vi "Main.vi"(11 "Module Admin":refnum<class "Delacor_lib_QMH_Module Admin.lvclass">) -> ()   [LabVIEW 2020, in "Motherboard loading.lvlib"]
doc: "This template is based off of the Queued Message Handler design pattern and the Queued Message Handler project template that ships with LabVIEW.\n\nThe main difference is that the queue is private to this module and communication between modules is performed via Broadcast and Request events.\n\nRequest events are wrapped in public API methods and are handled in the Event Handling Loop (EHL) of this VI. Any module can register for Broadcast events sent by this module. The EHL generates messages based on user interface actions.\n\nThe Message Handling Loop (MHL) processes messages generated by the EHL, or by other messages. The messages are string values, so new messages can be added easily to the Message Cases case structure in the MHL. Each message cluster can also provide an optional value for Message Data, which is a variant that can be converted to whatever message-specific data is required.\n_____\nBased on DQMH Project Template 6.1.0.94."
uses:
  Motherboard loading.lvlib
  <vilib>/Delacor/Delacor QMH/Libraries/Module Admin_class/Delacor_lib_QMH_Module Admin.lvclass
  Module Data--cluster.ctl
  <vilib>/Delacor/Delacor QMH/Libraries/Message Queue_class/Delacor_lib_QMH_Message Queue.lvclass/Delacor_lib_QMH_Message Queue.ctl
  Stop Argument--cluster.ctl
  <vilib>/Delacor/Delacor QMH/Libraries/Module Admin_class/Delacor_lib_QMH_Module Admin.lvclass/Delacor_lib_QMH_Module Admin.ctl
  Start acquisition Argument--cluster.ctl
  Start acquisition (Reply Payload)--cluster.ctl
  Stop acquisition Argument--cluster.ctl
  System.Management
  <vilib>/Utility/miscctls.llb/LVPointTypeDef.ctl
  <vilib>/Delacor/Delacor QMH/Libraries/Message Queue_class/Delacor_lib_QMH_Enqueue Message (Single).vi
  <vilib>/Delacor/Delacor QMH/Libraries/Module Admin_class/Delacor_lib_QMH_Get External Launch.vi
  <vilib>/Utility/error.llb/Error Cluster From Error Code.vi
  <vilib>/ErrorRing/Error Ring.xnode
  <vilib>/Delacor/Delacor QMH/Libraries/Message Queue_class/Delacor_lib_QMH_Message Queue.lvclass
panel:
  in  "format":i32(ring) items=["Mof", "CimDtd20", "WmiDtd20"]
  out "error out":errorcluster
  out "Status":string
  in  "Simulate MHL Error":bool
  in  "Simulate EHL Error":bool
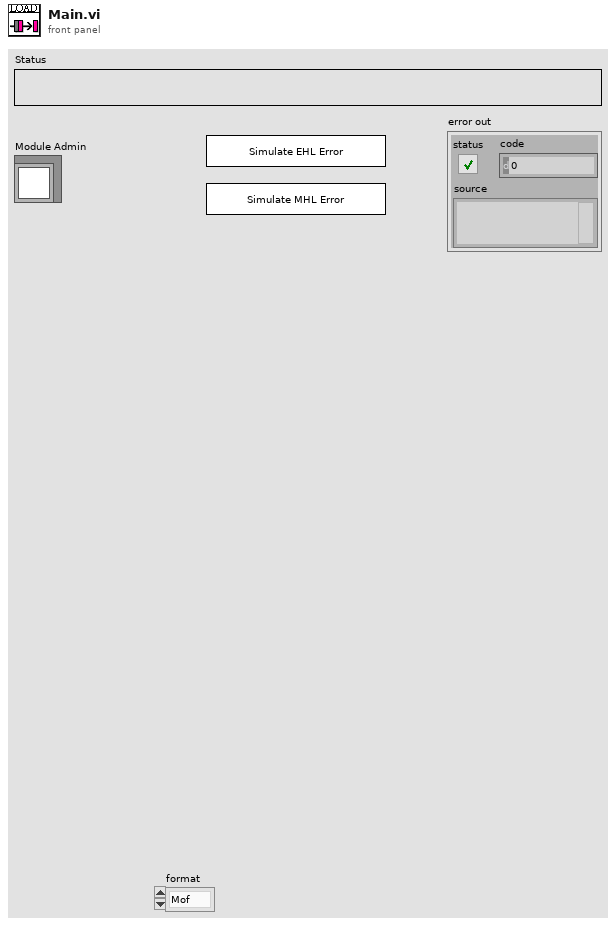
[diagram p1: front panel]
types:
  T1 = typedef "Motherboard loading.lvlib/Request Events--cluster.ctl" = cluster{"Stop Module":refnum<user-event>, "Show Panel":refnum<user-event>, "Hide Panel":refnum<user-event>, "Get Module Execution Status":refnum<user-event>, "Show Diagram":refnum<user-event>, "Start acquisition":refnum<user-event>, "Wake up Load detect HL":refnum<user-event>, "Put Load update HL to sleep":refnum<user-event>, "Stop acquisition":refnum<user-event>}
  T2 = typedef "Motherboard loading.lvlib/Module Data--cluster.ctl" = cluster{"Status":string}
  T3 = enum32{"invalid lock state", "Not Locked", "Locked (No Password)", "Password-protected"}
  T4 = typedef "Motherboard loading.lvlib/Stop Argument--cluster.ctl" = cluster{"Origin":string, "Exit via Stop Module Req?":bool, "Wait for Module to stop?":bool}
  T5 = typedef "Motherboard loading.lvlib/Start acquisition Argument--cluster.ctl" = cluster{"Boolean":bool, "Wait Notifier":refnum<notifier>, "wait for reply":bool, "Detecting speed":dbl}
  T6 = typedef "Motherboard loading.lvlib/Stop acquisition Argument--cluster.ctl" = cluster{"Boolean":bool}
  T7 = typedef "LVPointTypeDef.ctl" = cluster{"Horizontal":i16, "Vertical":i16}
  T8 = enum32{"Invalid", "Standard", "Closed", "Hidden", "Minimized", "Maximized"}
  T9 = typedef "Motherboard loading.lvlib/Start acquisition (Reply Payload)--cluster.ctl" = cluster{"error":errorcluster}
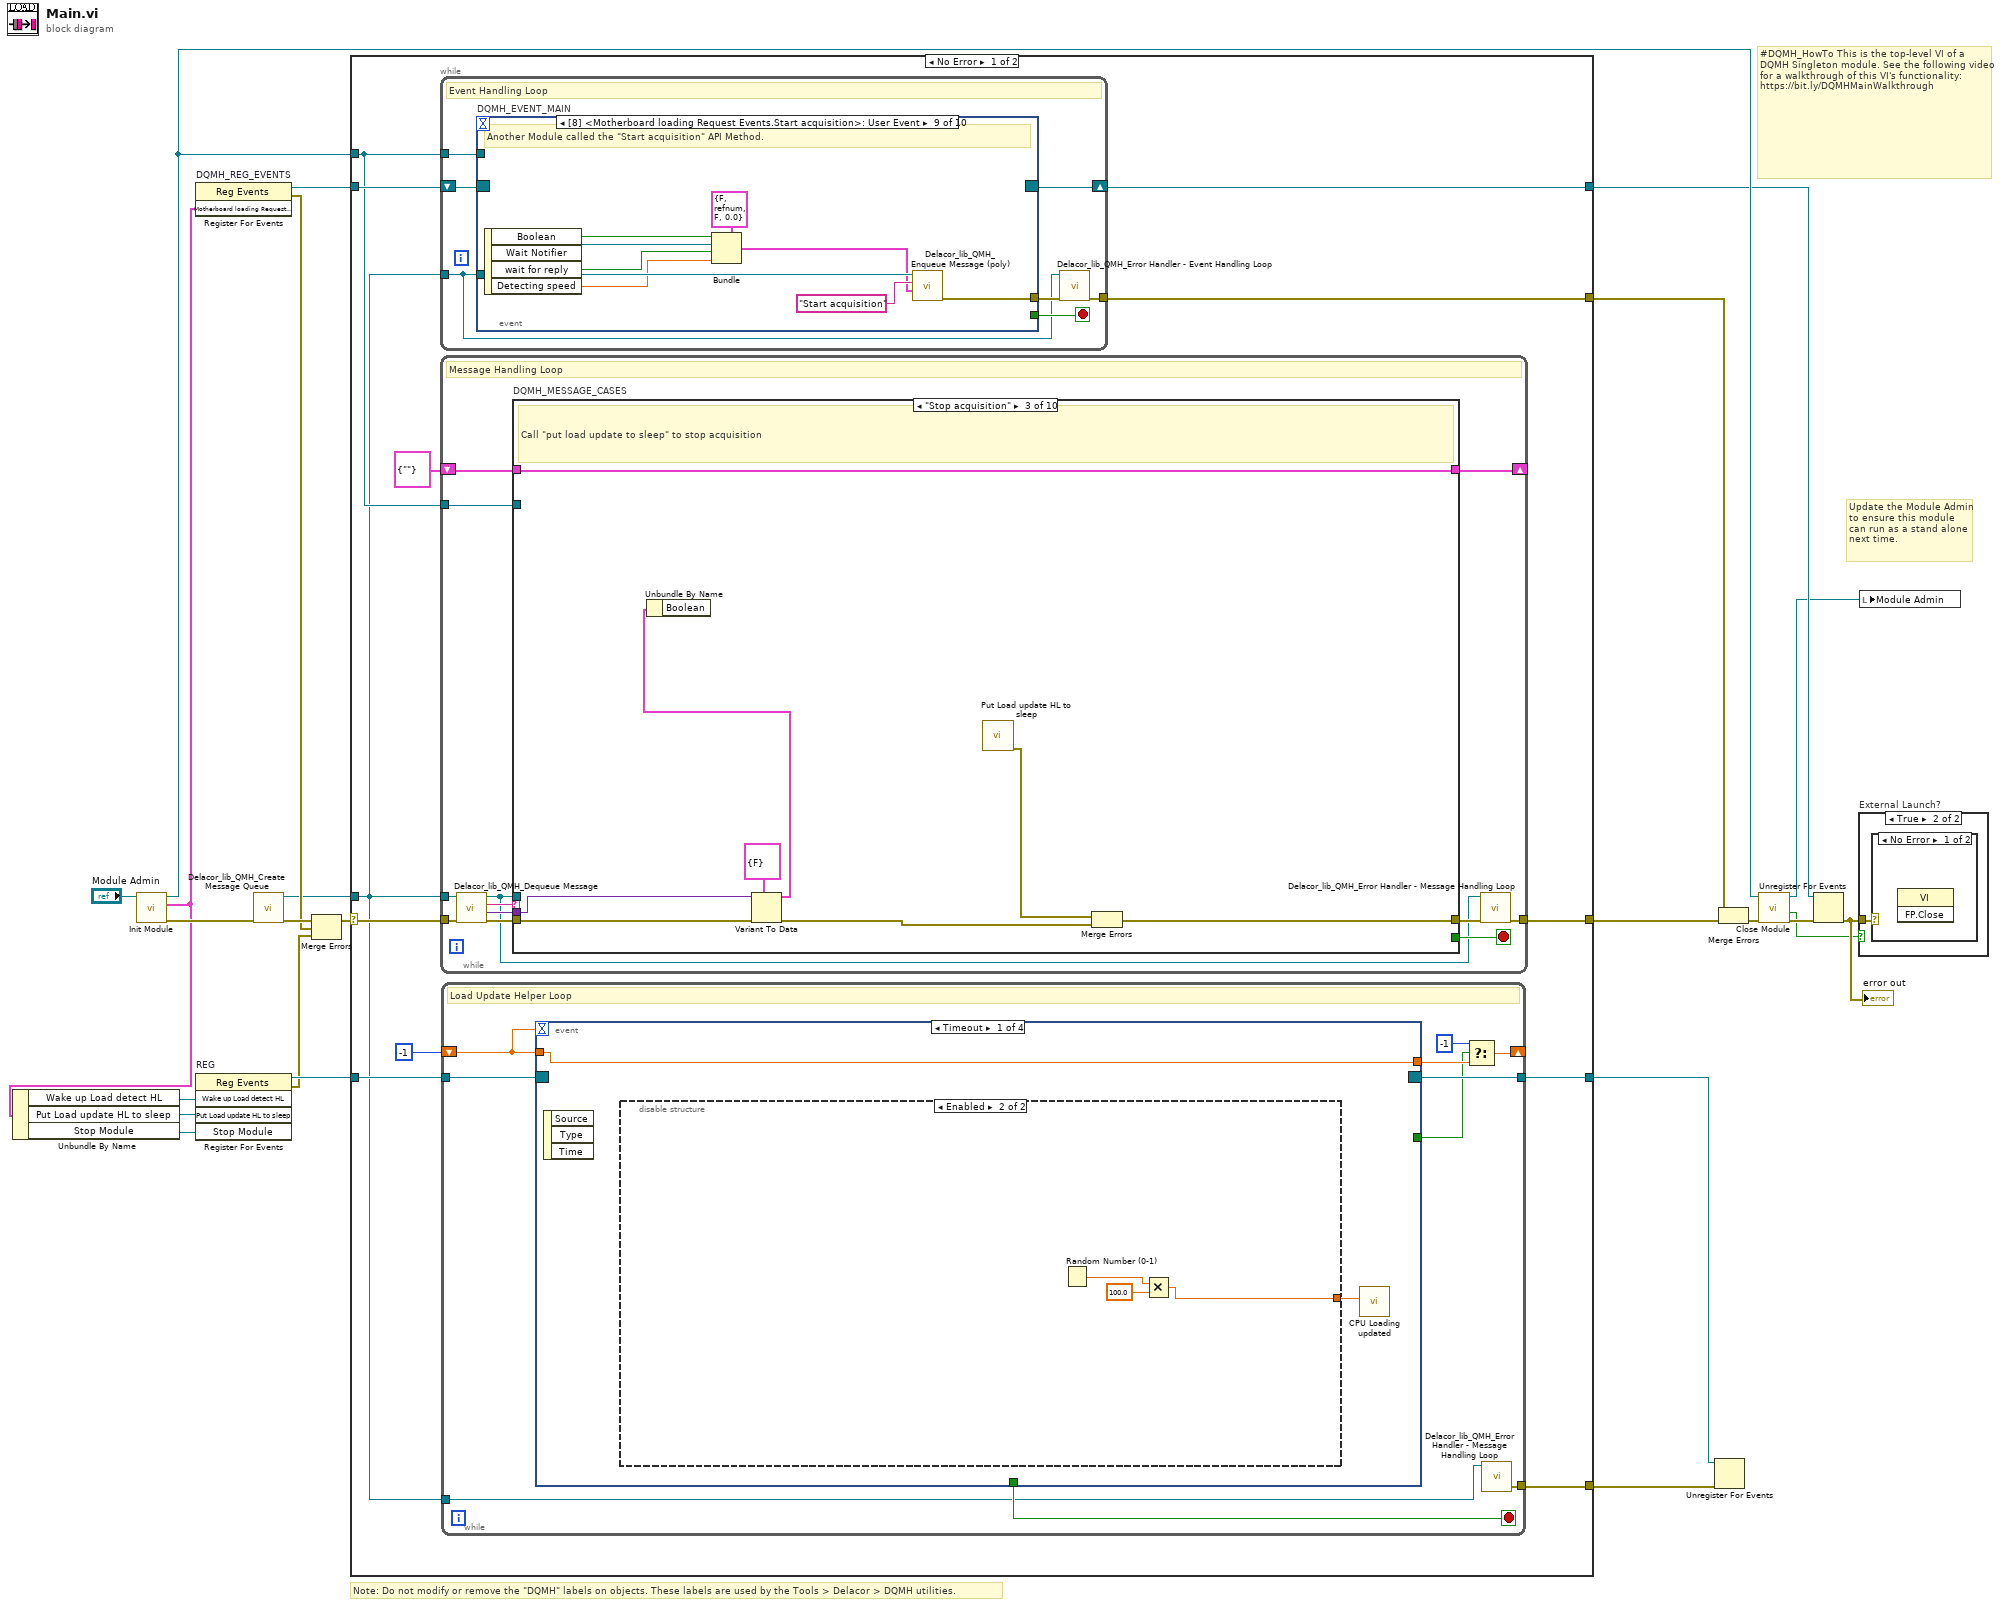
[diagram p0: block diagram]
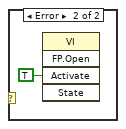
[diagram p3: hidden frame]
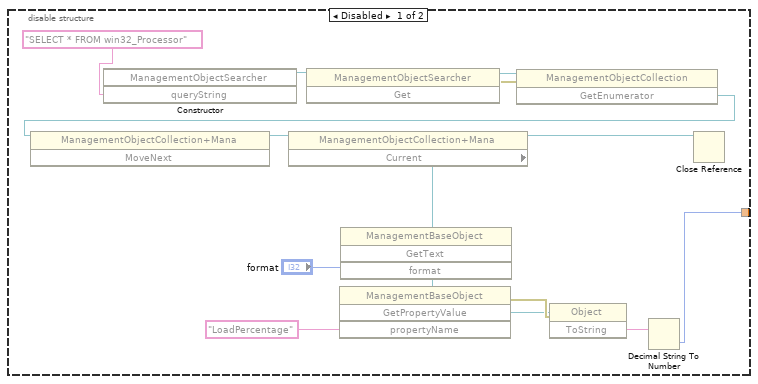
[diagram p4: hidden frame]
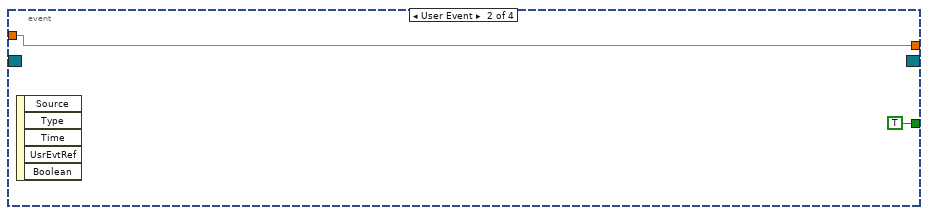
[diagram p5: hidden frame]
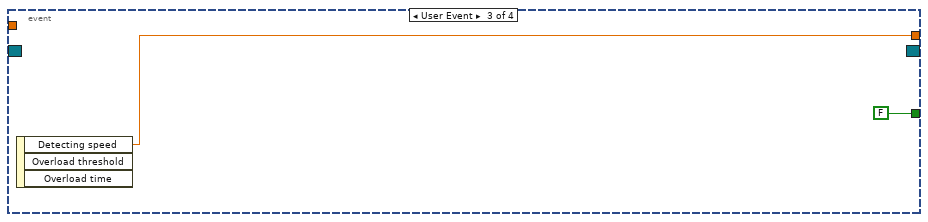
[diagram p6: hidden frame]
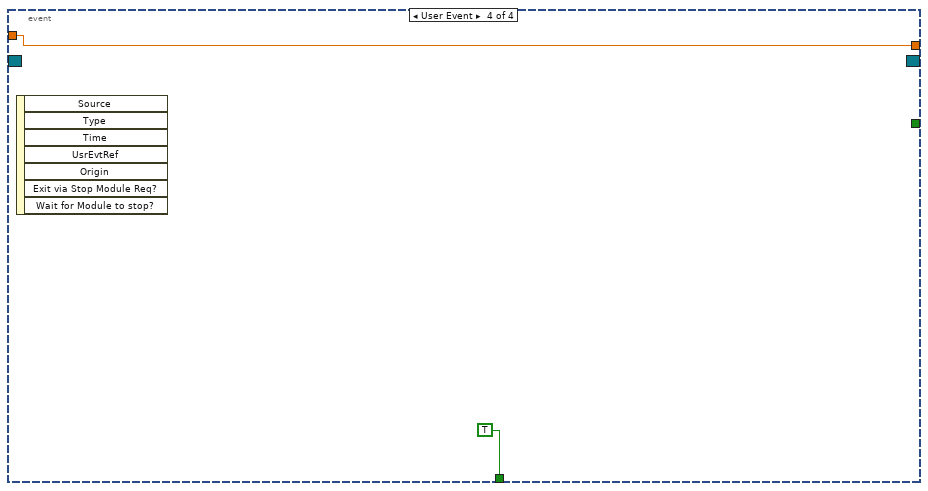
[diagram p7: hidden frame]
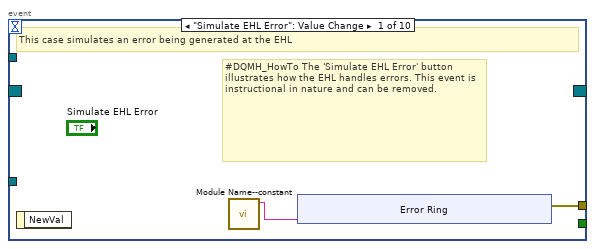
[diagram p8: hidden frame]
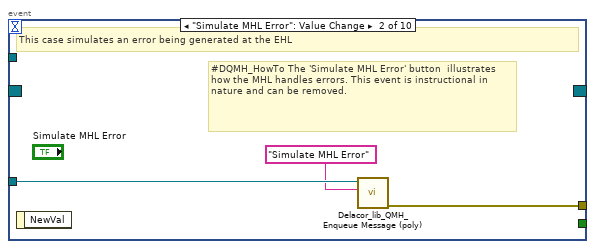
[diagram p9: hidden frame]
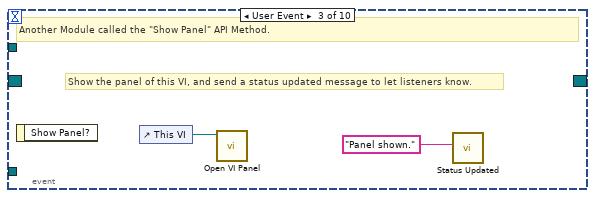
[diagram p10: hidden frame]
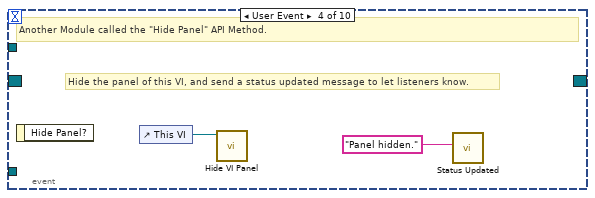
[diagram p11: hidden frame]
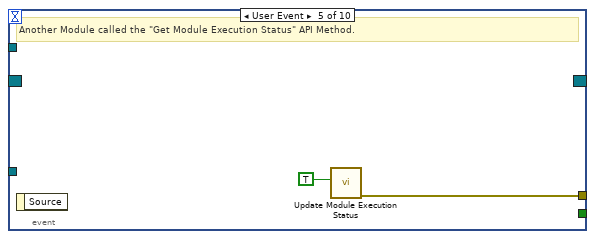
[diagram p12: hidden frame]
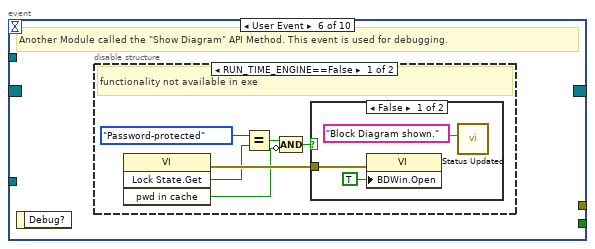
[diagram p13: hidden frame]
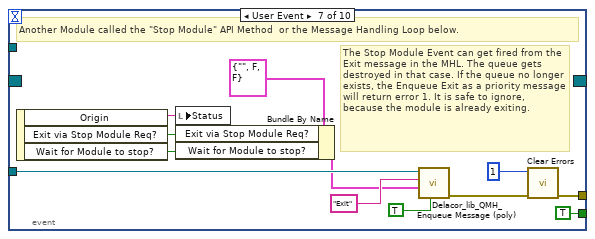
[diagram p16: hidden frame]
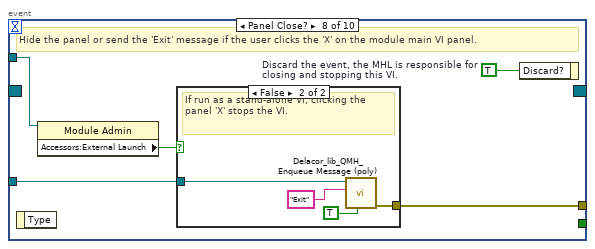
[diagram p17: hidden frame]
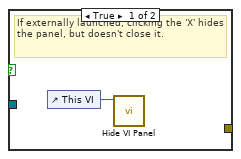
[diagram p18: hidden frame]
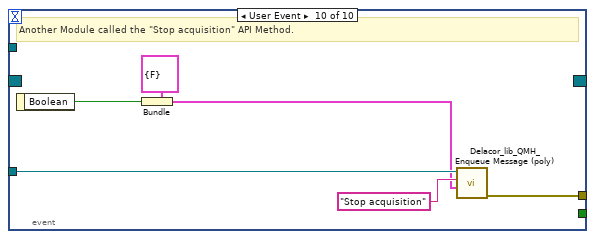
[diagram p19: hidden frame]
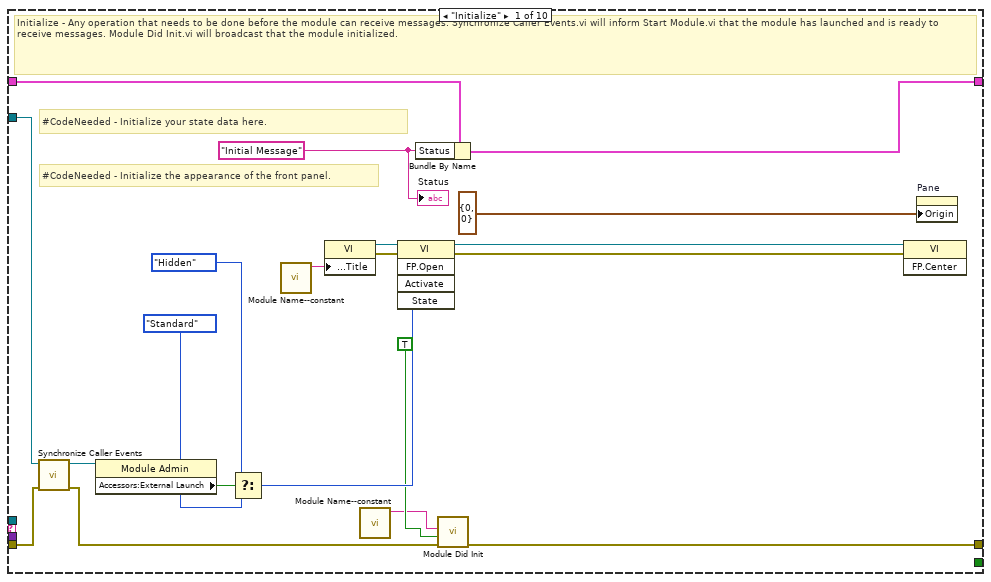
[diagram p20: hidden frame]
diagram:
  # "#DQMH_HowTo This is the top-level VI of a DQMH Singleton module. See the following video for a walkthrough of this VI's functionality: https://bit.ly/DQMHMainWalkthrough"
  # "Note: Do not modify or remove the \"DQMH\" labels on objects. These labels are used by the Tools > Delacor > DQMH utilities."
  # "Update the Module Admin to ensure this module can run as a stand alone next time."
  n1 = call "Init Module.vi"("Singleton Module Admin in"="Module Admin") -> ("error out"=w23:errorcluster, "Motherboard loading Request Events"=w2:T1, "Singleton Module Admin out"=w15:refnum<class "Delacor_lib_QMH_Module Admin.lvclass">)  [unwired: 8 in]
  n2 = Unbundle By Name(w2) -> ("Wake up Load detect HL"=w5:refnum<user-event>, "Put Load update HL to sleep"=w4:refnum<user-event>, "Stop Module"=w3:refnum<user-event>)
  n3 = register-events "DQMH_REG_EVENTS"(w2) -> (reference out=w13:refnum<event-registration>, error out=w16:errorcluster)  [unwired: 2 in]
  n4 = register-events "REG"(w5, w4, w3) -> (reference out=w8:refnum<event-registration>, error out=w1:errorcluster)  [unwired: 2 in]
  n5 = call <vilib>:"Delacor_lib_QMH_Create Message Queue.vi"("error in"=w23) -> ("error out"=w18:errorcluster, "Message Queue"=w12:refnum<class "Delacor_lib_QMH_Message Queue.lvclass">)  [unwired: 9 in]
  n6 = Merge Errors(w18, w16, w1) -> (w17:errorcluster)
  n7 = case shown="No Error" w17 {
    selector: w17 -> [w34 w267]
    tunnel: [w36 w266] -> w24
    tunnel: [w33 w272] -> w14
    tunnel: w13 -> [w31 w272]
    tunnel: w12 -> [w26 w265]
    tunnel: [w35 _] -> w21
    tunnel: w15 -> [w30 w268]
    tunnel: w8 -> [w29 w264]
    tunnel: [w28 _] -> w7
    tunnel: [w27 w264] -> w6
    frame No Error {
      n8 = while {
        tunnel: w26 -> [w72]
        shift-right: [w75] -> w33
        shift-left: w31 -> [w76]
        tunnel: [w77] -> w35
        tunnel: w30 -> [w73]
        stop <- w74 stop-if-true
        # "Event Handling Loop"
        n9 = event "DQMH_EVENT_MAIN" shown="[8] <Motherboard loading Request Events.Start acquisition>: User Event" {
          selector: w76 -> [_ _ _ _ _ _ _ _ _ _]
          dyn-events: [_ _ _ _ _ _ _ _ _ _] -> w75
          timeout: _ -> [_ _ _ _ _ _ _ _ _ _]
          tunnel: [_ _ _ _ _ _ TRUE ("Discard?") _ _ _] -> w74
          tunnel: w72 -> [_ w89 _ _ _ _ w113 w120 w136 w142]
          tunnel: [w80 w90 _ _ w96 _ w116 w122 w132 w137] -> w78
          tunnel: w73 -> [_ _ _ _ _ _ _ w119 _ _]
          event "Simulate EHL Error": Value Change {
            # "#DQMH_HowTo The 'Simulate EHL Error' button  illustrates how the EHL handles errors. This event is instructional in nature and can be removed."
            # "This case simulates an error being generated at the EHL"
            n10 = event-data() -> ()  [unwired: 1 in, 1 out]
            n11 = call "Module Name--constant.vi"() -> ("Module Name"=w79:string)  [unwired: 11 in]
            n12 = xnode "Error Ring"("parameter 0"=w79) -> ("error out"=w80:errorcluster)
          }
          event "Simulate MHL Error": Value Change {
            # "#DQMH_HowTo The 'Simulate MHL Error' button  illustrates how the MHL handles errors. This event is instructional in nature and can be removed."
            # "This case simulates an error being generated at the EHL"
            n13 = event-data() -> ()  [unwired: 1 in, 1 out]
            n14 = call-poly <vilib>:"Delacor_lib_QMH_Enqueue Message (poly).vi"("Message"="Simulate MHL Error", "Message Queue in"=w89) -> ("error out"=w90:errorcluster)  [unwired: 8 in, 1 out]
          }
          event User Event {
            # "Show the panel of this VI, and send a status updated message to let listeners know."
            # "Another Module called the \"Show Panel\" API Method."
            n15 = event-data() -> ()  [unwired: 1 in, 1 out]
            n16 = control-ref of="This VI"() -> (w92:refnum<vi>)
            n17 = call "Open VI Panel.vi"("VI"=w92) -> ()  [unwired: 10 in, 1 out]
            n18 = call "Status Updated.vi"("Status"="Panel shown." ("format string")) -> ()  [unwired: 10 in, 1 out]
          }
          event User Event {
            # "Hide the panel of this VI, and send a status updated message to let listeners know."
            # "Another Module called the \"Hide Panel\" API Method."
            n19 = event-data() -> ()  [unwired: 1 in, 1 out]
            n20 = control-ref of="This VI"() -> (w94:refnum<vi>)
            n21 = call "Hide VI Panel.vi"("VI"=w94) -> ()  [unwired: 10 in, 1 out]
            n22 = call "Status Updated.vi"("Status"="Panel hidden." ("format string")) -> ()  [unwired: 10 in, 1 out]
          }
          event User Event {
            # "Another Module called the \"Get Module Execution Status\" API Method."
            n23 = event-data() -> ()  [unwired: 1 in, 1 out]
            n24 = call "Update Module Execution Status.vi"("Running?"=TRUE) -> ("error out"=w96:errorcluster)  [unwired: 10 in]
          }
          event User Event {
            # "Another Module called the \"Show Diagram\" API Method. This event is used for debugging."
            n25 = event-data() -> ()  [unwired: 1 in, 1 out]
            n26 = disable-structure shown="RUN_TIME_ENGINE==False" {
              frame condition #0 (active) {
                # "functionality not available in exe"
                n27 = invoke class="VI" method="Lock State.Get"() -> (error out=w102:errorcluster, "Get Lock State"=w101:T3, "pwd in cache"=w98:bool)  [unwired: 4 in, 1 out]
                n28 = Equal?(x=T3."Password-protected", y=w101) -> (x = y?=w99:bool)
                n29 = Compound Arithmetic op=AND(w99, invert w98) -> (w97:bool)
                n30 = case shown="False" w97 {
                  tunnel: w102 -> [w105 _]
                  frame False {
                    n31 = property class="VI"(error in=w105, "BDWin.Open"=TRUE ("Block Diagram Window:Open")) -> ()  [unwired: 1 in, 2 out]
                    n32 = call "Status Updated.vi"("Status"="Block Diagram shown." ("format string")) -> ()  [unwired: 10 in, 1 out]
                  }
                  frame True {
                    # "Password-protected VI, and the password is not in the cache. Do not show the diagram."
                  }
                }
              }
              frame condition #1 {
              }
            }
          }
          event User Event {
            # "The Stop Module Event can get fired from the Exit message in the MHL. The queue gets destroyed in that case. If the queue no longer exists, the Enqueue Exit as a priority message will return error 1. It is safe to ignore, because the module is already exiting."
            # "Another Module called the \"Stop Module\" API Method  or the Message Handling Loop below."
            n33 = event-data() -> ("Origin"=w112:string, "Exit via Stop Module Req?"=w108:bool, "Wait for Module to stop?"=w107:bool)  [unwired: 1 in]
            n34 = local write "Status"(w112) -> ()
            n35 = Bundle By Name(cluster=T4 {"Origin"="", "Exit via Stop Module Req?"=FALSE, "Wait for Module to stop?"=FALSE} ("Stop Argument"), "Exit via Stop Module Req?"=w108, "Wait for Module to stop?"=w107) -> (w106:T4)
            n36 = call-poly <vilib>:"Delacor_lib_QMH_Enqueue Message (poly).vi"("Priority Message? (F)"=TRUE, "Message Data"=w106, "Message"="Exit", "Message Queue in"=w113) -> ("error out"=w117:errorcluster)  [unwired: 6 in, 1 out]
            n37 = call <vilib>:"Clear Errors.vi"("error in (no error)"=w117, "specific error code to clear (0: all)"=1) -> ("error out"=w116:errorcluster)  [unwired: 4 in, 1 out]
          }
          event Panel Close? {
            w121 = TRUE  # Discard the event, the MHL is responsible for closing and stopping this VI.
            # "Hide the panel or send the 'Exit' message if the user clicks the 'X' on the module main VI panel."
            n38 = event-data() -> ()  [unwired: 1 in, 1 out]
            n39 = property class="Module Admin"(reference=w119) -> ("Accessors:External Launch"=w118:bool)  [unwired: 1 in, 2 out]
            n40 = case shown="False" w118 {
              tunnel: w120 -> [_ w126]
              tunnel: [_ w127] -> w122
              frame True {
                # "If externally launched, clicking the 'X' hides the panel, but doesn't close it."
                n41 = control-ref of="This VI"() -> (w123:refnum<vi>)
                n42 = call "Hide VI Panel.vi"("VI"=w123) -> ()  [unwired: 10 in, 1 out]
              }
              frame False {
                # "If run as a stand-alone VI, clicking the panel 'X' stops the VI."
                n43 = call-poly <vilib>:"Delacor_lib_QMH_Enqueue Message (poly).vi"("Priority Message? (F)"=TRUE, "Message"="Exit", "Message Queue in"=w126) -> ("error out"=w127:errorcluster)  [unwired: 7 in, 1 out]
              }
            }
            n44 = event-data("Discard?"=w121) -> ()  [unwired: 1 in, 1 out]
          }
          event User Event {
            # "Another Module called the \"Start acquisition\" API Method."
            n45 = event-data() -> ("Boolean"=w131:bool, "Wait Notifier"=w130:refnum<notifier>, "wait for reply"=w129:bool, "Detecting speed"=w128:dbl)  [unwired: 1 in]
            n46 = Bundle(cluster=T5 {"Boolean"=FALSE, "Wait Notifier"=refnum, "wait for reply"=FALSE, "Detecting speed"=0.0} ("Start acquisition Argument"), "Boolean"=w131, "Wait Notifier"=w130, "wait for reply"=w129, "Detecting speed"=w128) -> (w133:T5)
            n47 = call-poly <vilib>:"Delacor_lib_QMH_Enqueue Message (poly).vi"("Message Data"=w133, "Message"="Start acquisition", "Message Queue in"=w136) -> ("error out"=w132:errorcluster)  [unwired: 7 in, 1 out]
          }
          event User Event {
            # "Another Module called the \"Stop acquisition\" API Method."
            n48 = event-data() -> ("Boolean"=w138:bool)  [unwired: 1 in]
            n49 = Bundle(cluster=T6 {"Boolean"=FALSE} ("Stop acquisition Argument"), "Boolean"=w138) -> (w139:T6)
            n50 = call-poly <vilib>:"Delacor_lib_QMH_Enqueue Message (poly).vi"("Message Data"=w139, "Message"="Stop acquisition", "Message Queue in"=w142) -> ("error out"=w137:errorcluster)  [unwired: 7 in, 1 out]
          }
        }
        n51 = call-dynamic "Delacor_lib_QMH_Error Handler - Event Handling Loop.vi"("error in"=w78, "Message Queue in"=w72) -> ("dup error in"=w77:errorcluster)  [unwired: 8 in, 1 out]
      }
      n52 = while {
        tunnel: w26 -> [w145]
        shift-right: [w149] -> _
        shift-left: T2 {"Status"=""} ("Data Cluster") -> [w150]
        tunnel: w34 -> [w153]
        tunnel: [w151] -> w36
        tunnel: w30 -> [w143]
        stop <- w148 stop-if-true
        # "Message Handling Loop"
        n53 = call-dynamic "Delacor_lib_QMH_Dequeue Message.vi"("error in"=w153, "Message Queue in"=w145) -> ("error out"=w152:errorcluster, "Message Data"=w146:variant, "Message"=w147:string, "Message Queue out"=w144:refnum<class "Delacor_lib_QMH_Message Queue.lvclass">)  [unwired: 6 in]
        n54 = case "DQMH_MESSAGE_CASES" shown="\"Stop acquisition\"" w147 {
          selector: w147 -> [_ _ _ _ _ _ _ _ _ w251]
          tunnel: w144 -> [_ _ _ _ _ _ _ w221 w243 _]
          tunnel: w152 -> [w172 w176 w184 w199 w204 w206 w211 w228 w249 w253]
          tunnel: [w170 w176 w179 w189 w203 w206 w210 w224 w246 w254] -> w154
          tunnel: w150 -> [w161 w175 w183 w198 w202 w205 w208 w223 w242 w252]
          tunnel: [w160 w175 w183 w198 w202 w205 w208 w223 w242 w252] -> w149
          tunnel: [_ _ _ _ _ _ _ _ w241 _] -> w148
          tunnel: w146 -> [_ _ w182 w196 _ _ _ w222 w240 _]
          tunnel: w143 -> [w162 _ _ _ _ _ _ w220 w235 _]
          frame "Initialize" {
            w156 = "Initial Message" ("Initial Message")
            # "#CodeNeeded - Initialize the appearance of the front panel."
            # "#CodeNeeded - Initialize your state data here."
            # "Initialize - Any operation that needs to be done before the module can receive messages. Synchronize Caller Events.vi will inform Start Module.vi that the module has launched and is ready to receive messages. Module Did Init.vi will broadcast that the module initialized."
            n55 = call "Synchronize Caller Events.vi"("error in (no error)"=w172, "Singleton Module Admin in"=w162) -> ("error out"=w171:errorcluster, "Singleton Module Admin out"=w157:refnum<class "Delacor_lib_QMH_Module Admin.lvclass">)  [unwired: 8 in]
            n56 = property class="Module Admin"(reference=w157) -> ("Accessors:External Launch"=w166:bool)  [unwired: 1 in, 2 out]
            n57 = Select(t=T8."Hidden" ("State"), s=w166, f=T8."Standard" ("State")) -> (s? t:f=w163:T8)
            n58 = call "Module Name--constant.vi"() -> ("Module Name"=w169:string)  [unwired: 11 in]
            n59 = property class="VI"("Front Panel.Title"=w169) -> (reference out=w168:refnum<vi>, error out=w174:errorcluster)  [unwired: 2 in]
            n60 = call "Module Name--constant.vi"() -> ("Module Name"=w158:string)  [unwired: 11 in]
            n61 = invoke class="VI" method="FP.Open"(reference=w168, error in=w174, "State"=w163) -> (reference out=w167:refnum<vi>, error out=w173:errorcluster)  [unwired: 2 in, 3 out]
            n62 = Bundle By Name(cluster=w161, "Status"=w156) -> (w160:T2)
            n63 = call "Module Did Init.vi"("error in (no error)"=w171, "Initialized?"=TRUE, "Origin"=w158) -> ("error out"=w170:errorcluster)  [unwired: 8 in]
            n64 = invoke class="VI" method="FP.Center"(reference=w167, error in=w173) -> ()  [unwired: 1 in, 3 out]
            n65 = property on="Pane" class="Pane"("Origin"=T7 {"Horizontal"=0, "Vertical"=0}) -> ()  [unwired: 2 in, 2 out]
            "Status" <- w156
          }
          frame "---Module Specific---" {
            # "Separator -- The following cases handle messages specific to this Module."
          }
          frame "Stop acquisition" {
            # "Call \"put load update to sleep\" to stop acquisition"
            n66 = Variant To Data(error in=w184, type=T6 {"Boolean"=FALSE} ("Stop acquisition Argument"), Variant=w182) -> (data=w180:T6, error out=w177:errorcluster)
            n67 = Unbundle By Name(w180) -> ()  [unwired: 1 out]
            n68 = call "Put Load update HL to sleep.vi"() -> ("error out"=w178:errorcluster)  [unwired: 11 in]
            n69 = Merge Errors(w178, w177) -> (w179:errorcluster)
          }
          frame "Start acquisition" {
            # "Reading processor usage percentage by wake up helper loop"
            n70 = Variant To Data(error in=w199, type=T5 {"Boolean"=FALSE, "Wait Notifier"=refnum, "wait for reply"=FALSE, "Detecting speed"=0.0} ("Start acquisition Argument"), Variant=w196) -> (data=w194:T5, error out=w197:errorcluster)
            n71 = Unbundle By Name(w194) -> ("Detecting speed"=w188:dbl, "Wait Notifier"=w193:refnum<notifier>, "wait for reply"=w192:bool)  [unwired: 1 out]
            n72 = call "Wake up Load detect HL.vi"("Overload time"=0.0, "Overload threshold"=0.0, "Detecting speed"=w188) -> ("error out"=w185:errorcluster)  [unwired: 8 in]
            n73 = Bundle By Name(cluster=T9 {"error"={"status"=FALSE, "code"=0, "source"=""}} ("Start acquisition (Reply Payload)"), "error"=w185) -> (w191:T9)
            n74 = Merge Errors(w197, w185) -> (w189:errorcluster)
            n75 = case "DQMH_FIRE_NOTIFIER" shown="True" w192 {
              tunnel: w193 -> [_ w201]
              tunnel: w191 -> [_ w200]
              frame False {
              }
              frame True {
                n76 = Send Notification(notification=w200, notifier=w201) -> ()  [unwired: 1 in, 2 out]
              }
            }
          }
          frame "---Copy This Frame---" {
            # "Duplicate this frame when creating new messages.  Change this comment in the duplicated frame to describe this message."
            n77 = Merge Errors(w204) -> (w203:errorcluster)
          }
          frame "---Exit and Error Handling---" {
            # "Separator - The following cases handle errors and exit messages."
          }
          frame "Simulate MHL Error" {
            # "#DQMH_HowTo The 'Simulate MHL Error' button  illustrates how the MHL handles errors. This event is instructional in nature and can be removed."
            # "Simulate an error occurring at the MHL"
            n78 = call "Module Name--constant.vi"() -> ("Module Name"=w207:string)  [unwired: 11 in]
            n79 = xnode "Error Ring"("parameter 0"=w207) -> ("error out"=w209:errorcluster)
            n80 = Merge Errors(w211, w209) -> (w210:errorcluster)
          }
          frame "Error" {
            # "#CodeRecommended - If you ever change the name of this \"Error\" message, you'll need to update the name in the Check Loop Error.vi as well."
            # "#CodeRecommended - If the module is running in standalone mode (External Launch = FALSE), this code will pop up an error dialog and call the 'Exit' message if an error occurs. Add more fine-grained error handling here."
            # "Error - Check the error message data and respond accordingly. This message is sent by the \"Error Handler\" VIs at the end of each loop in this application."
            n81 = property class="Module Admin"(reference=w220) -> ("Accessors:External Launch"=w219:bool)  [unwired: 1 in, 2 out]
            n82 = Variant To Data(error in=w228, type=errorcluster {"status"=FALSE, "code"=0, "source"=""} ("error constant"), Variant=w222) -> (data=w229:errorcluster, error out=w226:errorcluster)
            n83 = call "Error Reported.vi"("Error"=w229) -> ()  [unwired: 10 in, 1 out]
            n84 = case shown="False" w219 {
              tunnel: [w234 _] -> w225
              tunnel: w221 -> [w232 _]
              tunnel: w229 -> [w233 _]
              frame False {
                # "If the module is running standalone, then pop up an error dialog and call the \"Exit\" message."
                n85 = call <vilib>:"Simple Error Handler.vi"("error in (no error)"=w233) -> ()  [unwired: 4 in, 5 out]
                n86 = call-poly <vilib>:"Delacor_lib_QMH_Enqueue Message (poly).vi"("Priority Message? (F)"=TRUE, "Message"="Exit", "Message Queue in"=w232) -> ("error out"=w234:errorcluster)  [unwired: 7 in, 1 out]
              }
              frame True {
                # "If the module was launched externally, calling the Error Reported broadcast VI is the only action performed by the \"Error\" message. The module's caller can then process the error appropriately."
              }
            }
            n87 = Merge Errors(w226, w225) -> (w224:errorcluster)
            n88 = local write "error out"(w224) -> ()
          }
          frame "Exit" {
            w239 = 91  # 91: not all Exit messages will have an argument
            w241 = TRUE  # Stop the VI
            # "Release the message queue reference"
            # "#CodeNeeded - Add any required cleanup code here"
            # "Exit - Exit the application."
            n89 = Variant To Data(error in=w249, type=T4 {"Origin"="", "Exit via Stop Module Req?"=FALSE, "Wait for Module to stop?"=FALSE} ("Stop Argument"), Variant=w240) -> (data=w237:T4, error out=w245:errorcluster)
            n90 = call <vilib>:"Clear Errors.vi"("error in (no error)"=w245, "specific error code to clear (0: all)"=w239) -> ("error out"=w248:errorcluster)  [unwired: 4 in, 1 out]
            n91 = control-ref of="This VI"() -> (w236:refnum<vi>)
            n92 = call-dynamic "Delacor_lib_QMH_Release Message Queue.vi"("error in"=w248, "Message Queue"=w243) -> ("error out"=w247:errorcluster)  [unwired: 9 in]
            n93 = call "Handle Exit.vi"("Stop Argument"=w237, "Admin in"=w235, "VI reference"=w236) -> ("error out"=w244:errorcluster)  [unwired: 7 in, 1 out]
            n94 = Merge Errors(w247, w244) -> (w246:errorcluster)
          }
          frame Default {
            # "'Default' case only runs if there is a message that isn't defined in any of the other cases.  Output a programming error."
            n95 = call "Module Name--constant.vi"() -> ("Module Name"=w250:string)  [unwired: 11 in]
            n96 = xnode "Error Ring"("parameter 0"=w251, "parameter 1"=w250) -> ("error out"=w255:errorcluster)
            n97 = Merge Errors(w253, w255) -> (w254:errorcluster)
          }
        }
        n98 = call-dynamic "Delacor_lib_QMH_Error Handler - Message Handling Loop.vi"("error in"=w154, "Message Queue in"=w144) -> ("dup error in"=w151:errorcluster)  [unwired: 8 in, 1 out]
      }
      n99 = while {
        tunnel: w29 -> [w46]
        tunnel: [w38] -> w28
        tunnel: [w45] -> w27
        tunnel: w26 -> [w37]
        shift-right: [w42] -> _
        shift-left: -1 -> [w41]
        stop <- w44 stop-if-true
        # "Load Update Helper Loop"
        n100 = event shown="[0] Timeout" {
          selector: w46 -> [_ _ _ _]
          dyn-events: [_ _ _ _] -> w45
          timeout: w41 -> [_ _ _ _]
          tunnel: [_ _ _ TRUE] -> w44
          tunnel: w41 -> [w48 w67 _ w70]
          tunnel: [w48 w67 w68 w70] -> w40
          tunnel: [_ TRUE FALSE _] -> w39
          event Timeout {
            n101 = event-data() -> ()  [unwired: 1 in, 3 out]
            n102 = disable-structure shown="Enabled" {
              disable-tunnel: [w50 w63] -> w47
              frame Disabled {
                n103 = constructor class="ManagementObjectSearcher"("queryString"="SELECT * FROM win32_Processor") -> (reference out=w60:refnum<k24>)  [unwired: 3 in, 3 out]
                n104 = invoke class="ManagementObjectSearcher" method="Get"(reference=w60) -> (error out=w61:errorcluster, "Get"=w62:refnum<k24>)  [unwired: 2 in, 1 out]
                n105 = invoke class="ManagementObjectCollection" method="GetEnumerator"(reference=w62, error in=w61) -> ("GetEnumerator"=w59:refnum<k24>)  [unwired: 1 in, 2 out]
                n106 = invoke class="ManagementObjectCollection+Mana" method="MoveNext"(reference=w59) -> (reference out=w58:refnum<k24>)  [unwired: 2 in, 2 out]
                n107 = property class="ManagementObjectCollection+Mana"(reference=w58) -> (reference out=w52:refnum<k24>, "Current"=w53:refnum<k24>)  [unwired: 1 in, 1 out]
                n108 = invoke class="ManagementBaseObject" method="GetPropertyValue"(reference=w53, "propertyName"="LoadPercentage") -> (error out=w57:errorcluster, "GetPropertyValue"=w56:refnum<k24>)  [unwired: 2 in, 2 out]
                n109 = invoke class="ManagementBaseObject" method="GetText"(reference=w53, "format"="format") -> ()  [unwired: 2 in, 4 out]
                n110 = invoke class="Object" method="ToString"(reference=w56, error in=w57) -> ("ToString"=w51:string)  [unwired: 1 in, 2 out]
                n111 = Decimal String To Number(string=w51) -> (number=w50:i32)  [unwired: 2 in, 1 out]
                n112 = Close Reference(reference=w52) -> ()  [unwired: 1 in, 1 out]
              }
              frame Enabled {
                n113 = Random Number (0-1)() -> (number: 0 to 1=w64:dbl)
                n114 = Multiply(x=w64, y=100.0) -> (x*y=w63:dbl)
              }
            }
            n115 = call "CPU Loading updated.vi"("CPU Loading"=w47) -> ()  [unwired: 10 in, 1 out]
          }
          event User Event {
            n116 = event-data() -> ()  [unwired: 1 in, 5 out]
          }
          event User Event {
            n117 = event-data() -> ("Detecting speed"=w68:dbl)  [unwired: 1 in, 2 out]
          }
          event User Event {
            n118 = event-data() -> ()  [unwired: 1 in, 7 out]
          }
        }
        n119 = Select(t=-1, s=w39, f=w40) -> (s? t:f=w42:dbl)
        n120 = call-dynamic "Delacor_lib_QMH_Error Handler - Message Handling Loop.vi"("Message Queue in"=w37) -> ("dup error in"=w38:errorcluster)  [unwired: 9 in, 1 out]
      }
    }
    frame Error {
      # "Synchronize Caller Events.vi will inform Start Module.vi that the module has launched and will let the code calling Start Module.vi register for broadcasts and would permit the caller receive the broadcast that an error occurred at launch time."
      n121 = call-dynamic "Delacor_lib_QMH_Release Message Queue.vi"("error in"=w267, "Message Queue"=w265) -> ("error out"=w266:errorcluster)  [unwired: 9 in]
      n122 = call "Synchronize Caller Events.vi"("Singleton Module Admin in"=w268) -> ("error out"=w273:errorcluster)  [unwired: 9 in, 1 out]
      n123 = call "Module Name--constant.vi"() -> ("Module Name"=w271:string)  [unwired: 11 in]
      n124 = Format Into String(format string="An error occurred during initialization. %s is no longer running.", w271) -> (resulting string=w269:string)  [unwired: 2 in, 1 out]
      n125 = Merge Errors(w266, w273) -> (w274:errorcluster)
      n126 = call "Error Reported.vi"("Additional Information"=w269, "Error"=w274) -> ()  [unwired: 9 in, 1 out]
    }
  }
  n127 = Unregister For Events(event registration refnum=w6, error in=w7) -> ()  [unwired: 1 out]
  n128 = Merge Errors(w21, w24) -> (w20:errorcluster)
  n129 = call "Close Module.vi"("error in (no error)"=w20, "Module Admin in"=w15) -> ("error out"=w22:errorcluster, "External Launch"=w9:bool, "Module Admin out"=w10:refnum<class "Delacor_lib_QMH_Module Admin.lvclass">)  [unwired: 7 in]
  n130 = Unregister For Events(event registration refnum=w14, error in=w22) -> (error out=w19:errorcluster)
  "error out" <- w19
  n131 = case "External Launch?" shown="True" w9 {
    tunnel: w19 -> [_ w275]
    frame False {
    }
    frame True {
      n132 = case shown="No Error" w275 {
        frame No Error {
          n133 = invoke class="VI" method="FP.Close"() -> ()  [unwired: 3 in, 3 out]
        }
        frame Error {
          n134 = invoke class="VI" method="FP.Open"("Activate"=TRUE ("Activate?")) -> ()  [unwired: 4 in, 5 out]
        }
      }
    }
  }
  n135 = local write "Module Admin"(w10) -> ()
